vi "Toff.vi"(5 "preset time (ms)":i32=1000, 7 "input":bool, 11 "error in":errorcluster) -> (6 "off":u8, 8 "elapsed time (ms)":i32, 15 "error out":errorcluster)   [LabVIEW 2022 SP3, in "BinarySignalProcessClass.lvclass"]
uses:
  BinarySignalProcessClass.lvclass
  <vilib>/functionblocks/Counter/Timer Off Delay/Timer Off Delay.vi
  <vilib>/functionblocks/FB Core/FB Core.xnode
  BinarySignalProcessClass.lvclass/BinarySignalProcessClass.ctl
  <vilib>/functionblocks/NI_FunctionBlock Libraries.lvlib
  <vilib>/functionblocks/Edge Detection/Edge Detect/Edge Detect.vi
  <vilib>/functionblocks/Counter/Pulse Timer/Pulse Timer.vi
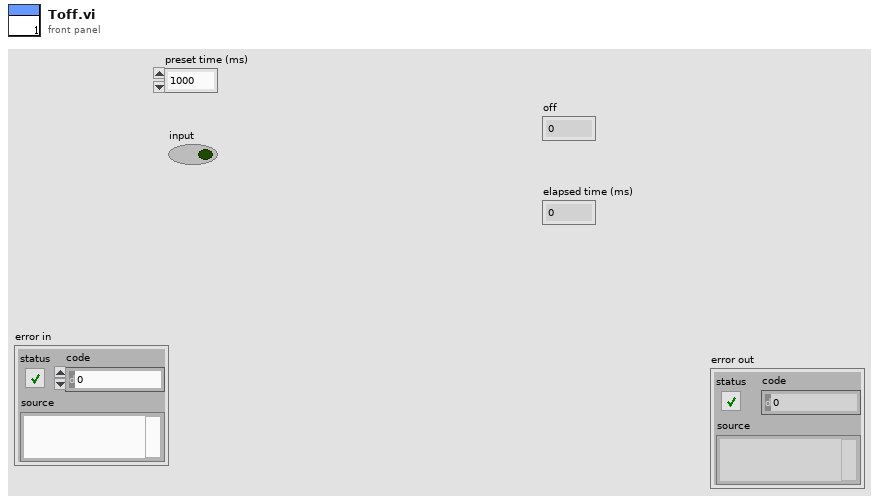
[diagram p1: front panel]
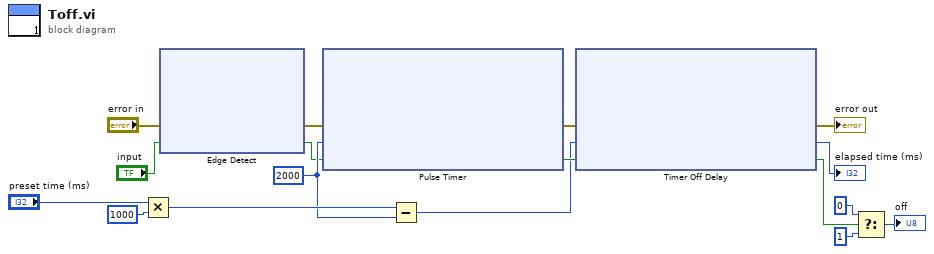
[diagram p0: block diagram]
diagram:
  w6 = 2000 ("preset time (ms)")
  n1 = Multiply(x="preset time (ms)", y=1000) -> (x*y=w7:i32)
  n2 = xnode "Edge Detect"("error in"="error in", "input 2"="input") -> ("error out"=w2:errorcluster, "output"=w1:bool)
  n3 = xnode "Pulse Timer"("error in"=w2, "preset time (ms)"=w6, "input"=w1) -> ("error out"=w8:errorcluster, "output"=w9:bool)  [unwired: 1 out]
  n4 = Subtract(x=w7, y=w6) -> (x-y=w5:i32)
  n5 = xnode "Timer Off Delay"("error in"=w8, "preset time (ms)"=w5, "input"=w9) -> ("error out"=→"error out":errorcluster, "elapsed time (ms)"=→"elapsed time (ms)":i32, "output"=w16:bool)
  n6 = Select(t=u8 0, s=w16, f=u8 1 ("t")) -> (s? t:f=→"off":u8)
